vi "setup_sections.vi"(8 "Error In":errorcluster) -> (0 "Error Out":errorcluster, 3 "Parameters Array":T2[](array[typedef]))   [LabVIEW 2019]
doc: "Setup the sections to analyze and the parameters used for each."
uses:
  section_parameters_cluster_typedef.ctl
  sections_method_enum_typedef.ctl
  sections_edge_mode_enum_typedef.ctl
  sections_roi_size_enum_typedef.ctl
  xi_angles_enum_typedef.ctl
  setup_sections_states_enum_typedef.ctl
panel:
  out "Section":T1(plugin-control)
  out "Sections to Analyze":string[](array[string])
  in  "Done":bool
  in  "Add":bool
  in  "Section Parameters":T2
  # "Set Section Analysis Parameters"
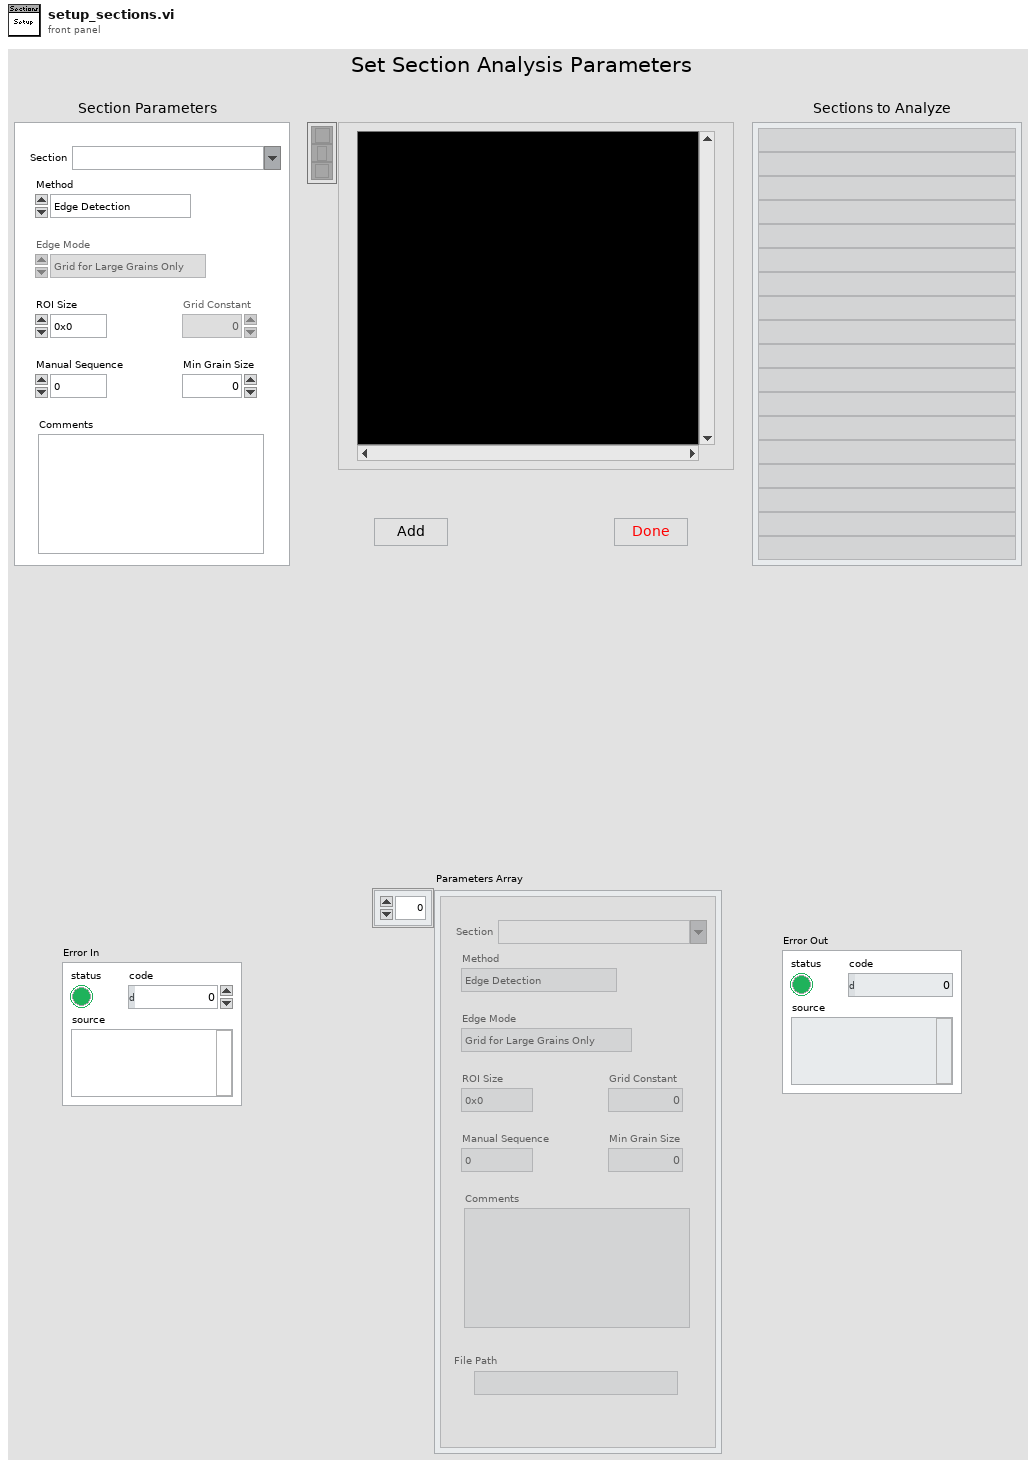
[diagram p1: front panel]
types:
  T1 = typedef "IMAQ Image.ctl" = refnum<image>
  T2 = typedef "section_parameters_cluster_typedef.ctl" = cluster{"Section":string, "Method":T3, "Edge Mode":T4, "ROI Size":T5, "Manual Sequence":T6, "Grid Constant":i32, "Min Grain Size":dbl, "Comments":string, "File Path":path}
  T3 = typedef "sections_method_enum_typedef.ctl" = enum16{"Edge Detection", "Grid Only", "Manual Selection", "Existing Edges"}
  T4 = typedef "sections_edge_mode_enum_typedef.ctl" = enum16{"Grid for Large Grains Only", "Grid", "No Grid"}
  T5 = typedef "sections_roi_size_enum_typedef.ctl" = enum16{"0x0", "1x1", "2x2", "3x3", "4x4", "5x5", "6x6"}
  T6 = typedef "xi_angles_enum_typedef.ctl" = enum16{"0", "45"}
  T7 = typedef "setup_sections_states_enum_typedef.ctl" = enum16{"Initialize", "Shutdown", "Add Section", "Update Control Visibility", "Wait", "Change Image"}
  T8 = enum8{"Enabled", "Disabled", "Disabled and Grayed Out"}
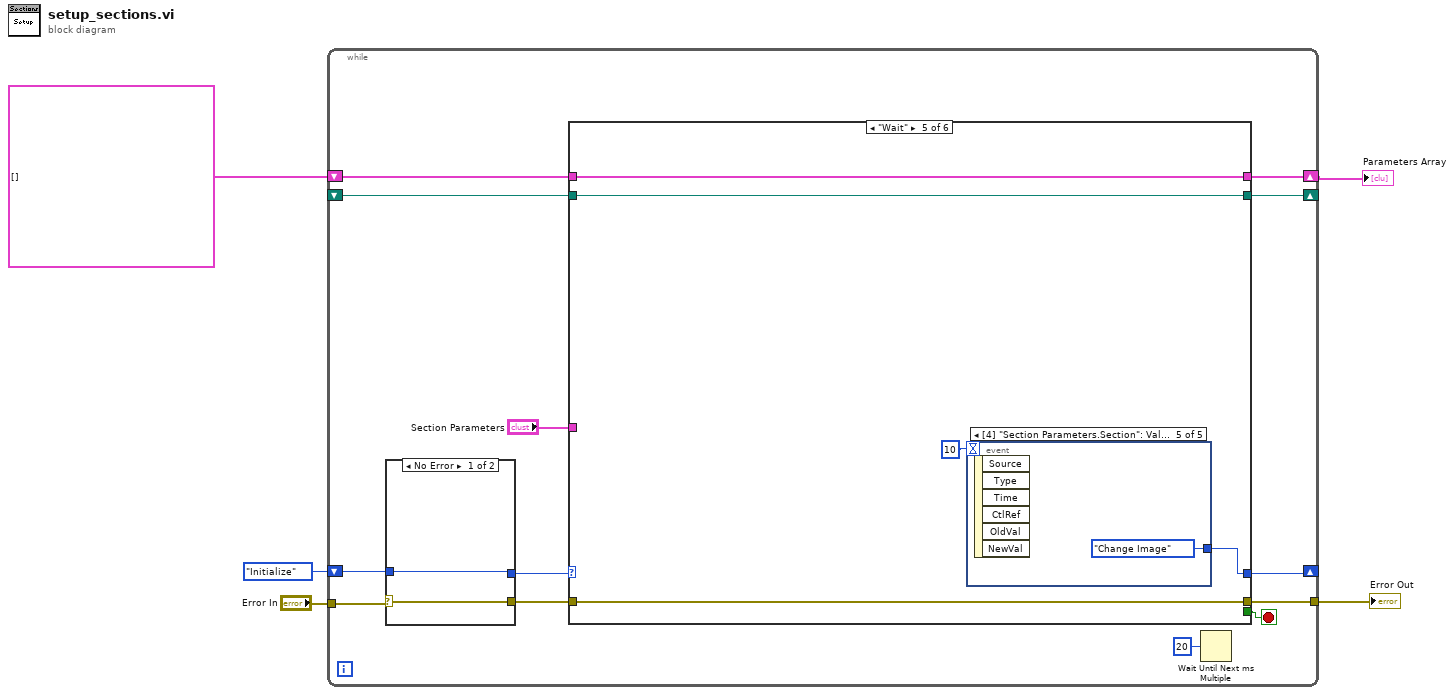
[diagram p0: block diagram]
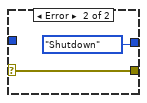
[diagram p2: hidden frame]
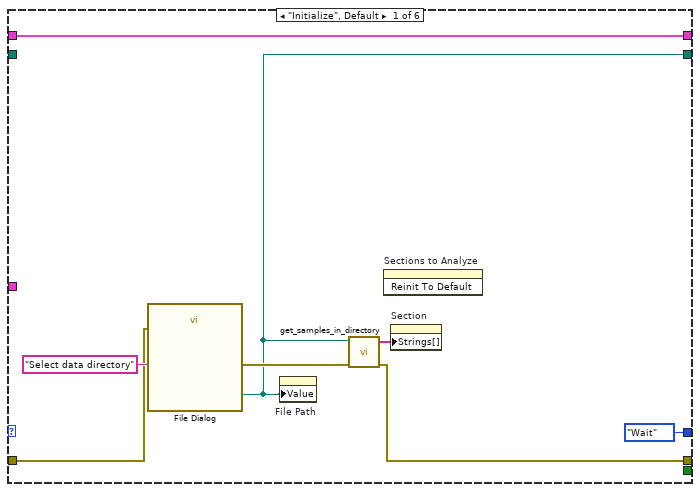
[diagram p3: hidden frame]
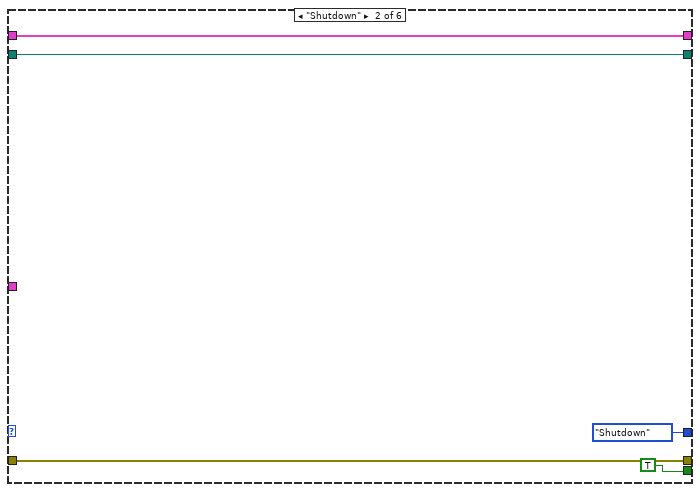
[diagram p4: hidden frame]
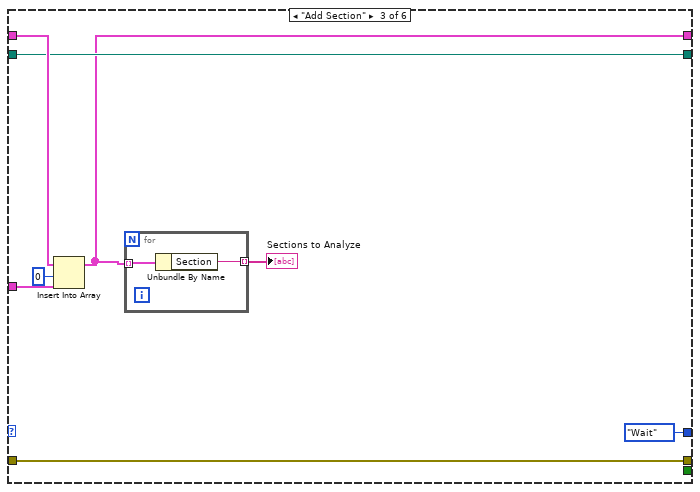
[diagram p5: hidden frame]
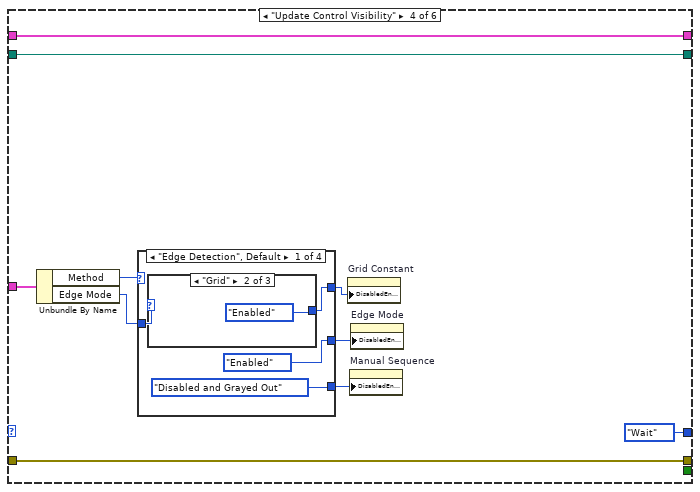
[diagram p6: hidden frame]
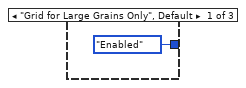
[diagram p7: hidden frame]
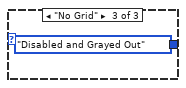
[diagram p8: hidden frame]
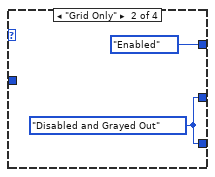
[diagram p9: hidden frame]
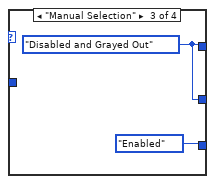
[diagram p10: hidden frame]
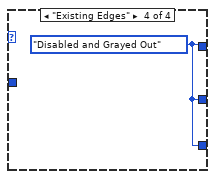
[diagram p11: hidden frame]
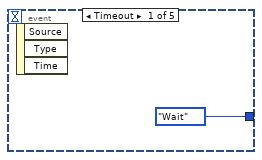
[diagram p12: hidden frame]
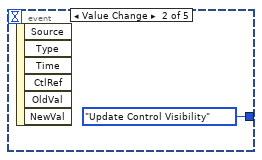
[diagram p13: hidden frame]
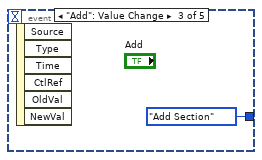
[diagram p14: hidden frame]
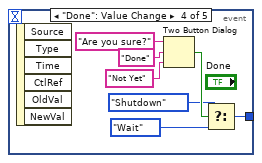
[diagram p15: hidden frame]
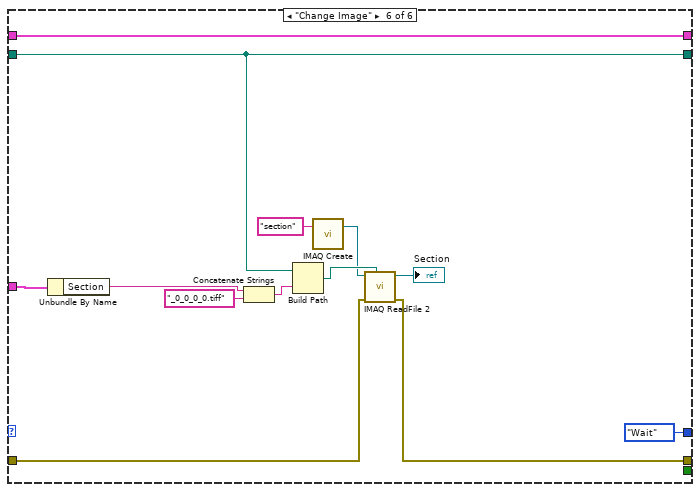
[diagram p16: hidden frame]
diagram:
  n1 = while {
    tunnel: "Error In" -> [w18]
    tunnel: [w14] -> w3
    shift-right: [w13] -> _
    shift-left: setup_sections_states_enum_typedef."Initialize" -> [w17]
    shift-right: [w10] -> w1
    shift-left: T2[] [] ("Parameters Array") -> [w9]
    shift-right: [w8] -> _
    shift-left: _ -> [w7]
    stop <- w12 stop-if-true
    n2 = case shown="No Error" w18 {
      selector: w18 -> [w19 w21]
      tunnel: [w20 setup_sections_states_enum_typedef."Shutdown"] -> w16
      tunnel: w17 -> [w20 _]
      tunnel: [w19 w21] -> w15
      frame No Error {
      }
      frame Error {
      }
    }
    n3 = case shown="\"Wait\"" w16 {
      tunnel: w15 -> [w27 w35 w39 w46 w72 w92]
      tunnel: [w24 w35 w39 w46 w72 w87] -> w14
      tunnel: [setup_sections_states_enum_typedef."Wait" setup_sections_states_enum_typedef."Shutdown" setup_sections_states_enum_typedef."Wait" setup_sections_states_enum_typedef."Wait" w70 setup_sections_states_enum_typedef."Wait"] -> w13
      tunnel: [_ TRUE _ _ _ _] -> w12
      tunnel: [w30 w32 w37 w55 w69 w96] -> w10
      tunnel: w9 -> [w30 w32 w42 w55 w69 w96]
      tunnel: [w25 w31 w40 w54 w68 w94] -> w8
      tunnel: w7 -> [_ w31 w40 w54 w68 w94]
      tunnel: "Section Parameters" -> [_ _ w38 w53 _ w95]
      frame "Initialize", Default {
        n4 = call "File Dialog"("prompt"="Select data directory", "error in"=w27) -> ("selected path"=w25:path, "error out"=w26:errorcluster)  [unwired: 10 in, 2 out]
        n5 = property on="File Path" class="Path"("Value"=w25) -> ()  [unwired: 2 in, 2 out]
        n6 = call "get_samples_in_directory.vi"("Error In"=w26, "Data Directory"=w25) -> ("Error Out"=w24:errorcluster, "Samples"=w23:string[])  [unwired: 8 in]
        n7 = invoke on="Sections to Analyze" class="Arr (strict)" method="Reinit To Default"() -> ()  [unwired: 3 in, 3 out]
        n8 = property on="Section" class="CmbBox"("Strings[]"=w23) -> ()  [unwired: 2 in, 2 out]
      }
      frame "Shutdown" {
      }
      frame "Add Section" {
        n9 = Insert Into Array(array=w42, index=0, new element=w38) -> (w37:T2[])
        n10 = for {
          tunnel: w37 -> [w45] mode=indexing
          tunnel: [w44] -> w36 mode=indexing
          n11 = Unbundle By Name(w45) -> ("Section"=w44:string)
        }
        "Sections to Analyze" <- w36
      }
      frame "Update Control Visibility" {
        n12 = Unbundle By Name(w53) -> ("Method"=w52:T3, "Edge Mode"=w51:T4)
        n13 = case shown="\"Edge Detection\", Default" w52 {
          tunnel: w51 -> [w59 _ _ _]
          tunnel: [w58 T8."Enabled" ("Disabled") w66 w67] -> w50
          tunnel: [T8."Enabled" ("Disabled") w63 w66 w67] -> w49
          tunnel: [T8."Disabled and Grayed Out" ("Disabled") w63 T8."Enabled" ("Disabled") w67] -> w48
          frame "Edge Detection", Default {
            n14 = case shown="\"Grid\"" w59 {
              tunnel: [T8."Enabled" ("Disabled") T8."Enabled" ("Disabled") T8."Disabled and Grayed Out" ("Disabled")] -> w58
              frame "Grid for Large Grains Only", Default {
              }
              frame "Grid" {
              }
              frame "No Grid" {
              }
            }
          }
          frame "Grid Only" {
            w63 = T8."Disabled and Grayed Out" ("Disabled")
          }
          frame "Manual Selection" {
            w66 = T8."Disabled and Grayed Out" ("Disabled")
          }
          frame "Existing Edges" {
            w67 = T8."Disabled and Grayed Out" ("Disabled")
          }
        }
        n15 = property on="Grid Constant" class="DigNum (strict)"("DisabledEnum"=w50) -> ()  [unwired: 2 in, 2 out]
        n16 = property on="Manual Sequence" class="Enum (strict)"("DisabledEnum"=w48) -> ()  [unwired: 2 in, 2 out]
        n17 = property on="Edge Mode" class="Enum (strict)"("DisabledEnum"=w49) -> ()  [unwired: 2 in, 2 out]
      }
      frame "Wait" {
        n18 = event shown="[4] \"Section Parameters.Section\": Value Change" {
          selector: _ -> [_ _ _ _ _]
          dyn-events: _ -> [_ _ _ _ _]
          timeout: 10 -> [_ _ _ _ _]
          tunnel: [setup_sections_states_enum_typedef."Wait" setup_sections_states_enum_typedef."Update Control Visibility" setup_sections_states_enum_typedef."Add Section" w76 setup_sections_states_enum_typedef."Change Image"] -> w70
          event Timeout {
            n19 = event-data() -> ()  [unwired: 1 in, 3 out]
          }
          event Value Change {
            n20 = event-data() -> ()  [unwired: 1 in, 6 out]
          }
          event "Add": Value Change {
            n21 = event-data() -> ()  [unwired: 1 in, 6 out]
          }
          event "Done": Value Change {
            n22 = event-data() -> ()  [unwired: 1 in, 6 out]
            n23 = Two Button Dialog(message="Are you sure?", 1:"Not Yet" ("F button name (\"Cancel\")"), 2:"Done" ("T button name (\"OK\")")) -> (T button?=w79:bool)
            n24 = Select(t=setup_sections_states_enum_typedef."Shutdown", s=w79, f=setup_sections_states_enum_typedef."Wait") -> (s? t:f=w76:T7)
          }
          event Value Change {
            n25 = event-data() -> ()  [unwired: 1 in, 6 out]
          }
        }
      }
      frame "Change Image" {
        n26 = Unbundle By Name(w95) -> ("Section"=w90:string)
        n27 = Concatenate Strings(w90, "_0_0_0_0.tiff" ("string")) -> (w91:string)
        n28 = Build Path(base path=w94, name or relative path=w91) -> (appended path=w93:path)
        n29 = call "IMAQ Create"("Image Name"="section") -> ("New Image"=w84:T1)  [unwired: 4 in, 1 out]
        n30 = call "IMAQ ReadFile 2"("File Path"=w93, "error in (no error)"=w92, "Image"=w84) -> ("error out"=w87:errorcluster, "Image Out"=→"Section":T1)  [unwired: 4 in, 3 out]
      }
    }
    n31 = Wait Until Next ms Multiple(millisecond multiple=u32 20) -> ()  [unwired: 1 out]
  }
  "Error Out" <- w3
  "Parameters Array" <- w1
